vi "TEST 2.vi"() -> ()   [LabVIEW 2014, in "SetUp VIs.lvlib"]
uses:
  SetUp VIs.lvlib
panel:
  out "text":string
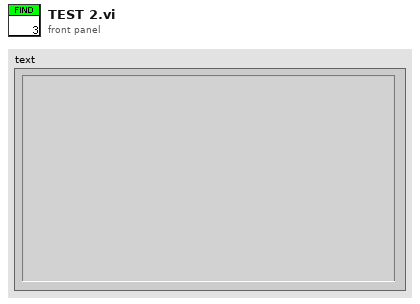
[diagram p1: front panel]
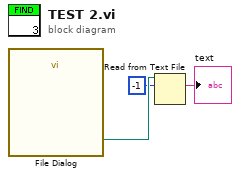
[diagram p0: block diagram]
diagram:
  n1 = call "File Dialog"() -> ("selected path"=w2:path)  [unwired: 12 in, 3 out]
  n2 = Read from Text File(file (use dialog)=w2, count=-1) -> (text=→"text":string)  [unwired: 2 in, 3 out]
